vi "String_Find Any Pattern Match.vi"(7 "Start Index (0)":i32, 10 "Target":string, 11 "Target List":string[](array[string])) -> (2 "Exact Match Out":bool, 3 "Index Out":i32)   [LabVIEW 2020]
uses:
  daaa9eff-712e-497d-ae34-0a6b443bd322.vi
  b6a16de6-4b00-4e98-8248-8915008b39a1.vi
  daaa9eff-712e-497d-ae34-0a6b443bd322.vi/1eead1fb-27fb-4f9c-8207-3c02e4fa65d6.vi
  b6a16de6-4b00-4e98-8248-8915008b39a1.vi/b5e579bd-ac25-4342-ba81-b7284c6f1874.vi
  <vilib>/Utility/error.llb/Trim Whitespace.vi
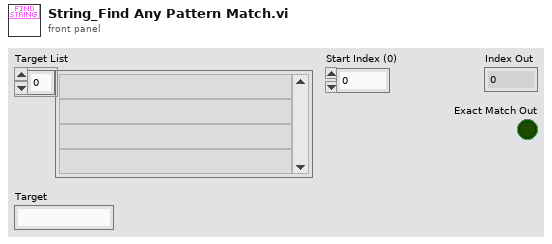
[diagram p1: front panel]
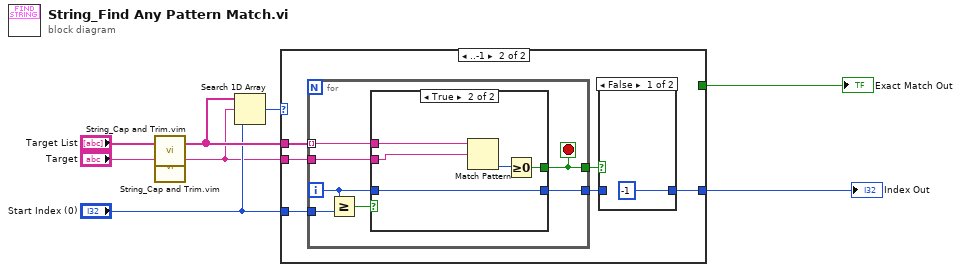
[diagram p0: block diagram]
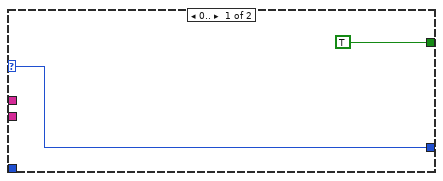
[diagram p2: hidden frame]
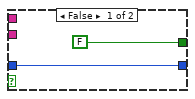
[diagram p4: hidden frame]
diagram:
  n1 = call "String_Cap and Trim.vim"("String In"="Target List") -> ("String Array Out"=w7:string[])  [unwired: 2 in]
  n2 = call "String_Cap and Trim.vim"("String In"="Target") -> ("String Array Out"=w3:string)  [unwired: 2 in]
  n3 = Search 1D Array(1D array=w7, element=w3, start index (0)="Start Index (0)") -> (index of element=w6:i32)
  n4 = case shown="..-1" w6 {
    selector: w6 -> [w10 _]
    tunnel: "Start Index (0)" -> [_ w16]
    tunnel: [w10 w14] -> w8
    tunnel: w3 -> [_ w12]
    tunnel: w7 -> [_ w11]
    tunnel: [TRUE _] -> w4
    frame 0.. {
    }
    frame ..-1 {
      n5 = for {
        tunnel: w11 -> [w19] mode=indexing
        tunnel: w12 -> [w25]
        tunnel: [w20] -> w13
        tunnel: [w24] -> w15
        tunnel: w16 -> [w23]
        i -> [w21]
        stop <- w24 stop-if-true
        n6 = Greater Or Equal?(x=w21, y=w23) -> (x >= y?=w22:bool)
        n7 = case shown="True" w22 {
          tunnel: w19 -> [_ w32]
          tunnel: w25 -> [_ w31]
          tunnel: [FALSE w29] -> w24
          tunnel: w21 -> [w26 w28]
          tunnel: [w26 w28] -> w20
          frame False {
          }
          frame True {
            n8 = Match Pattern(string=w32, regular expression=w31) -> (offset past match=w30:i32)  [unwired: 1 in, 3 out]
            n9 = Greater Or Equal To 0?(x=w30) -> (x >= 0?=w29:bool)
          }
        }
      }
      n10 = case shown="False" w15 {
        tunnel: w13 -> [_ w18]
        tunnel: [-1 w18] -> w14
        frame False {
        }
        frame True {
        }
      }
    }
  }
  "Index Out" <- w8
  "Exact Match Out" <- w4
